vi "press and sound.vi"(9 "stop":bool) -> (10 "frequency":dbl, 11 "data":dbl)   [LabVIEW 2019]
uses:
  <vilib>/sound2/lvsound2.llb/Sound Data Format.ctl
  <vilib>/sound2/lvsound2.llb/Sampling Mode.ctl
  <vilib>/sound2/lvsound2.llb/Sound Output Set Volume (Single).vi
  <vilib>/sound2/lvsound2.llb/Sound Output Write (DBL Single).vi
panel:
  out "0, 1":i16
  out "Array":bool[][](array[boolean])=[[FALSE, FALSE, TRUE, FALSE, FALSE, FALSE, TRUE, FALSE, FALSE, FALSE], [TRUE, TRUE, FALSE, TRUE, FALSE, TRUE, TRUE, FALSE, FALSE, FALSE], [FALSE, TRUE, TRUE, TRUE, FALSE, TRUE, TRUE, FALSE, FALSE, FALSE], [FALSE, FALSE, TRUE, TRUE, TRUE, FALSE, TRUE, FALSE, FALSE, FALSE], [FALSE, TRUE, TRUE, TRUE, TRUE, TRUE, FALSE, FALSE, FALSE, FALSE], [TRUE, TRUE, TRUE, TRUE, TRUE, TRUE, FALSE, FALSE, FALSE, FALSE], [FALSE, FALSE, TRUE, FALSE, FALSE, TRUE, TRUE, TRUE, TRUE, TRUE], [TRUE, TRUE, TRUE, TRUE, TRUE, TRUE, TRUE, TRUE, TRUE, TRUE], [FALSE, TRUE, TRUE, TRUE, TRUE, TRUE, TRUE, TRUE, TRUE, TRUE]]
  in  "stop 4":bool
  out "Boolean":bool
  out "Boolean 5":bool
  out "Boolean 4":bool
  out "Boolean 7":bool
  out "Boolean 6":bool
  out "Boolean 2":bool
  out "Boolean 3":bool
  out "Boolean 8":bool
  out "Boolean 9":bool
  out "Boolean 10":bool
  out "Boolean 11":bool
  out "Boolean 12":bool
  out "Boolean 13":bool
  out "Boolean 14":bool
  out "output array":bool[](array[boolean])
  out "data 8":bool[](array[boolean]) caption="data"
  in  "stop 3":bool
  out "score":dbl
  out "press7":dbl
  out "press6":dbl
  out "press5":dbl
  out "press4":dbl
  out "press3":dbl
  out "press2":dbl
  out "press":dbl
  out "ARDUINO7":dbl
  out "ARDUINO6":dbl
  out "ARDUINO5":dbl
  out "ARDUINO4":dbl
  out "ARDUINO3":dbl
  out "ARDUINO2":dbl
  out "ARDUINO":dbl
  in  "stop (T)":bool=TRUE
  out "data 7":dbl
  out "data 6":dbl
  out "data 5":dbl
  out "data 4":dbl
  out "data 3":dbl
  in  "stop (F) 2":bool caption="stop (F)"
  out "data 2":dbl
  in  "stop 2":bool
  out "Waveform Chart":waveform(dbl)(graph)
  in  "volume":dbl(slide) scale=0.0..100.0
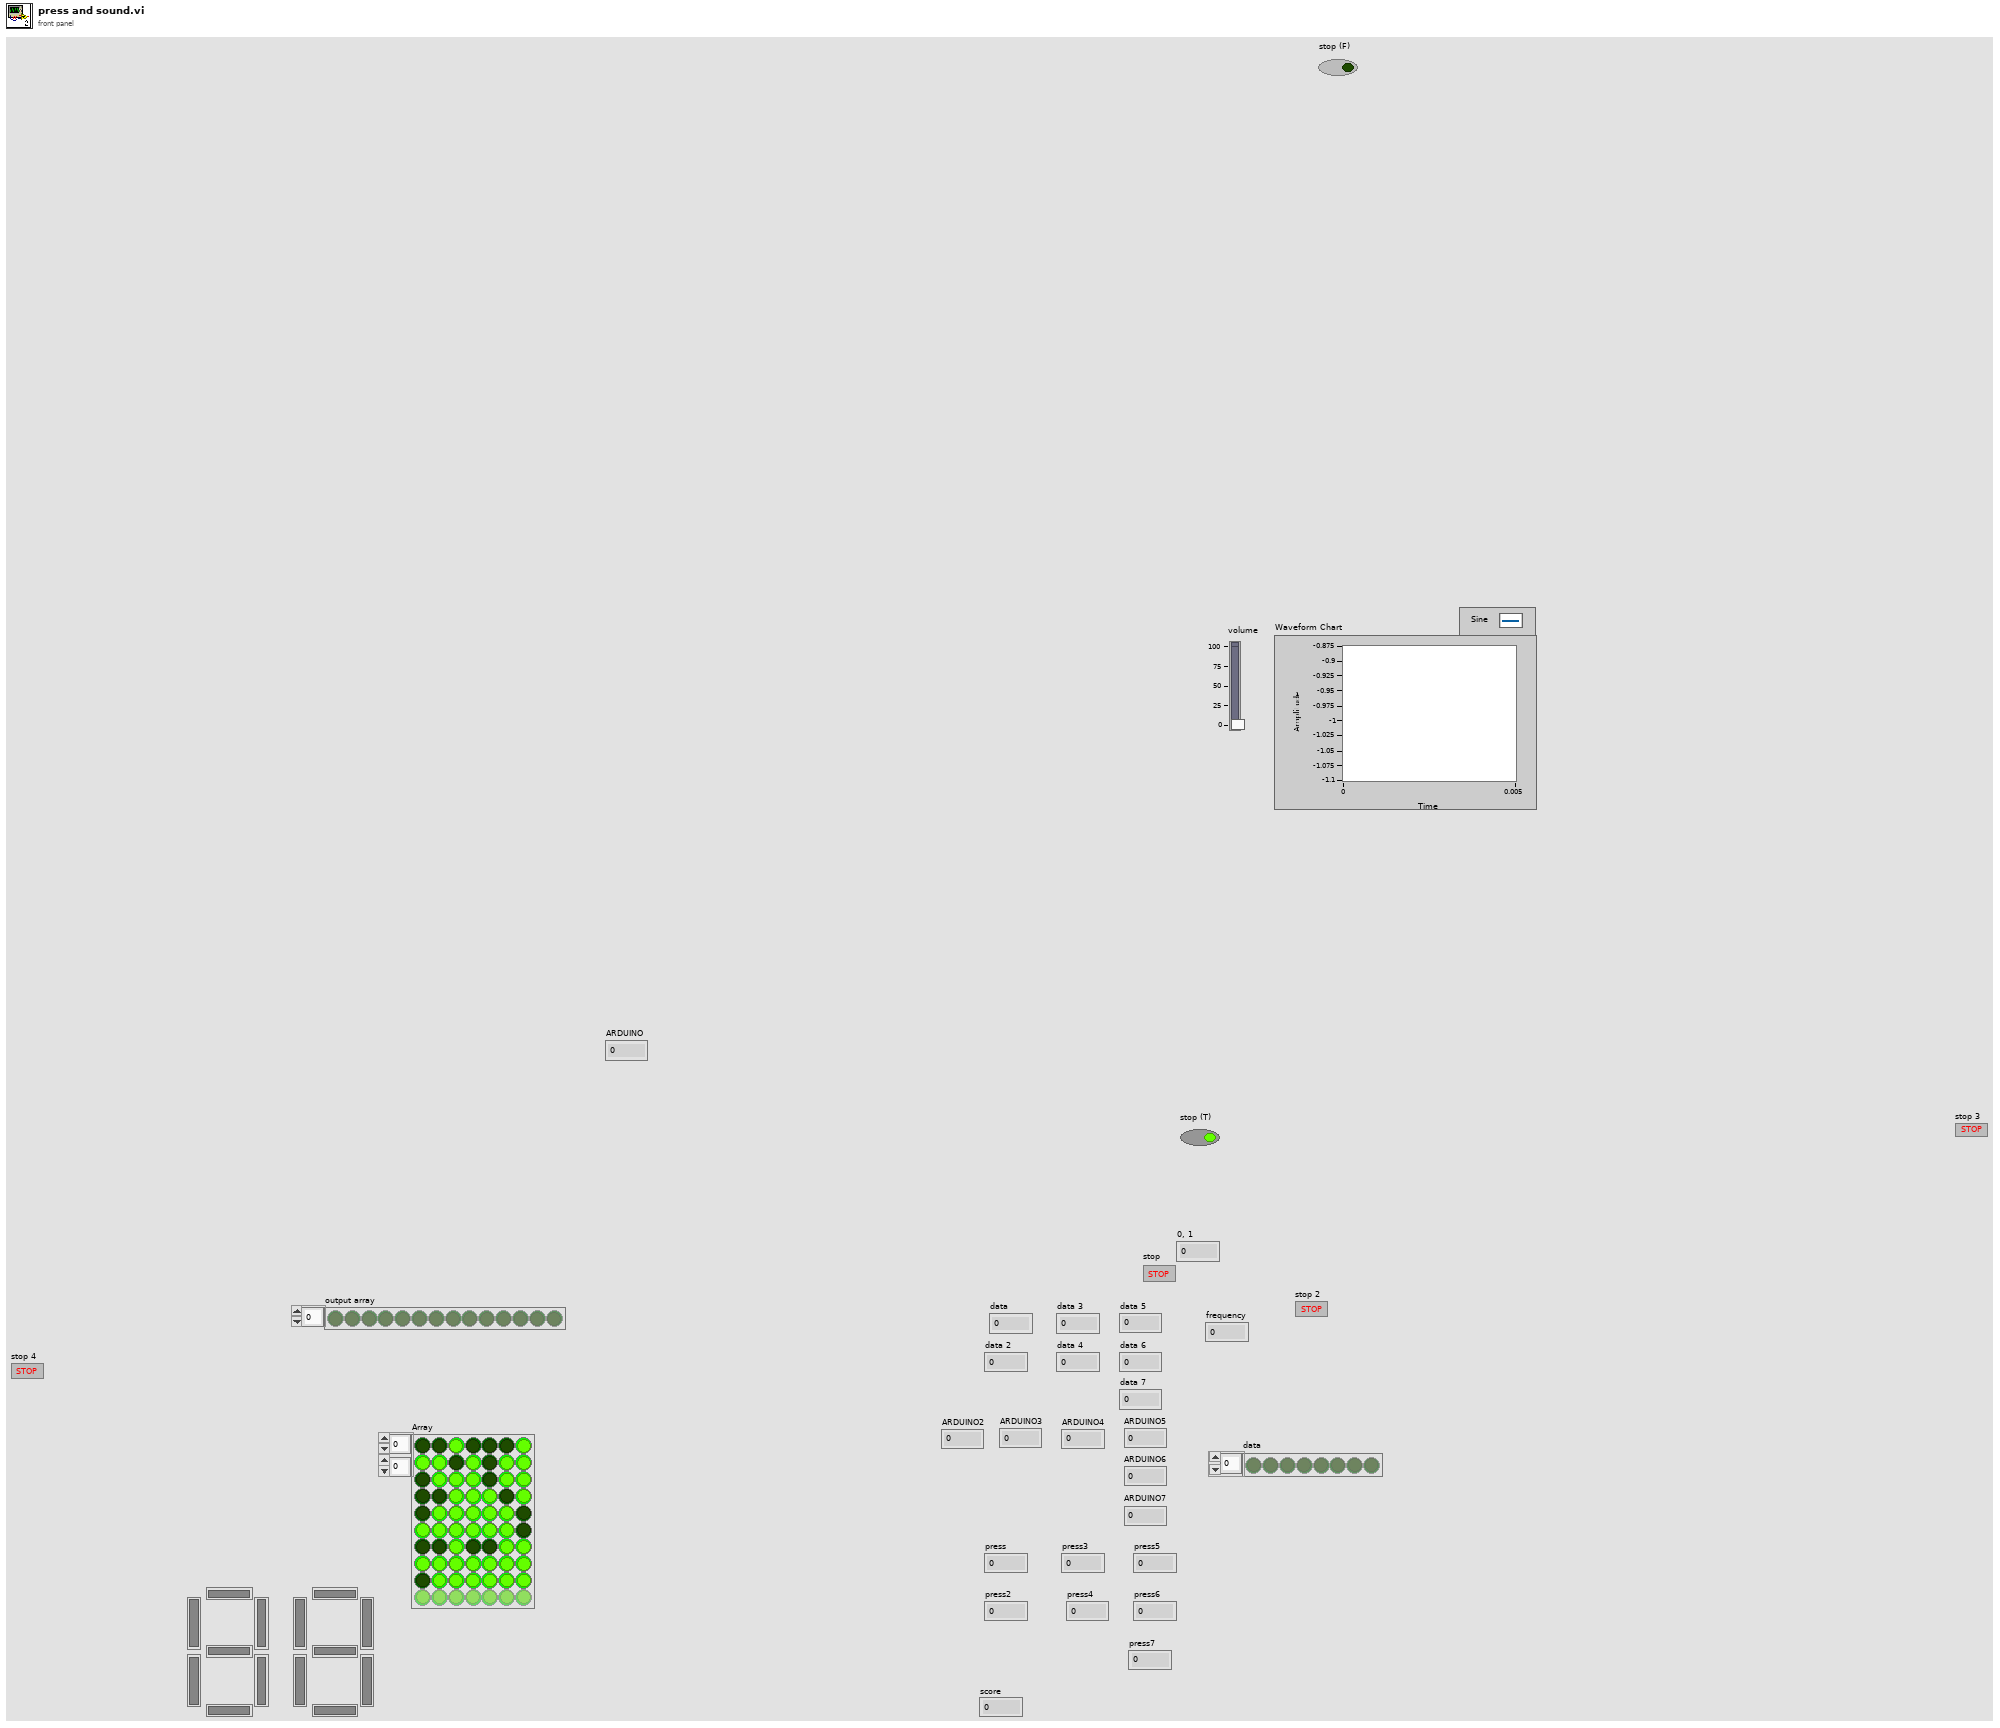
[diagram p1: front panel]
types:
  T1 = typedef "Sampling Mode.ctl" = i32
  T2 = typedef "Sound Data Format.ctl" = cluster{"sample rate (S/s)":dbl, "number of channels":i32, "bits per sample":i32}
  T3 = typedef "Sound Output Task ID.ctl" = u32
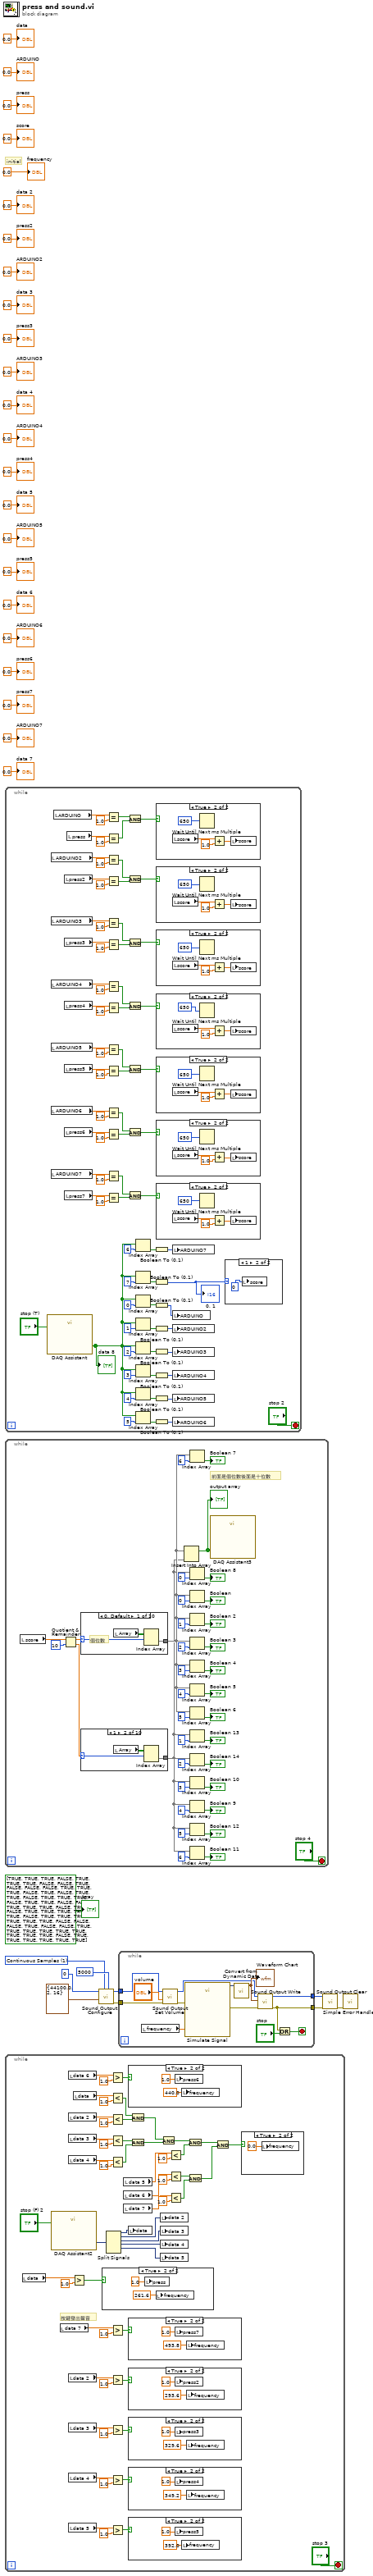
[diagram p0: block diagram]
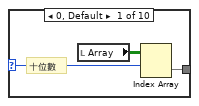
[diagram p2: hidden frame]
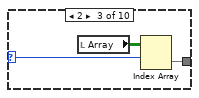
[diagram p3: hidden frame]
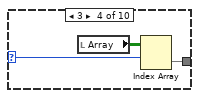
[diagram p4: hidden frame]
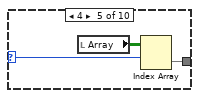
[diagram p5: hidden frame]
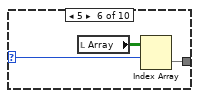
[diagram p6: hidden frame]
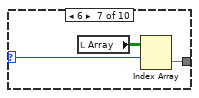
[diagram p7: hidden frame]
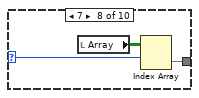
[diagram p8: hidden frame]
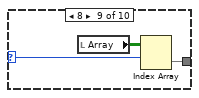
[diagram p9: hidden frame]
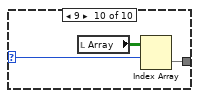
[diagram p10: hidden frame]
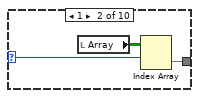
[diagram p11: hidden frame]
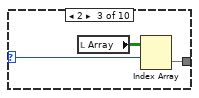
[diagram p12: hidden frame]
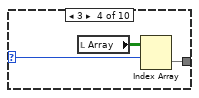
[diagram p13: hidden frame]
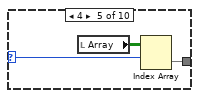
[diagram p14: hidden frame]
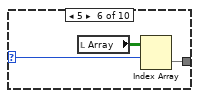
[diagram p15: hidden frame]
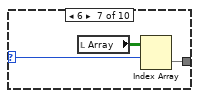
[diagram p16: hidden frame]
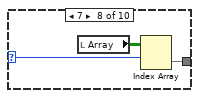
[diagram p17: hidden frame]
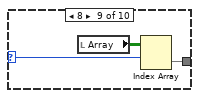
[diagram p18: hidden frame]
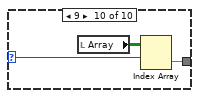
[diagram p19: hidden frame]
diagram:
  w25 = T1 1 items=["Finite Samples", "Continuous Samples"] ("sample mode")
  # "initial"
  n1 = while {
    stop <- "stop 2" stop-if-true
    n2 = call "DAQ Assistant"("stop (T)"="stop (T)") -> ("data"=w36:bool[])  [unwired: 16 in, 2 out]
    "data 8" <- w36
    n3 = local read "ARDUINO2"() -> (w105:dbl)
    n4 = local read "ARDUINO3"() -> (w103:dbl)
    n5 = local read "ARDUINO4"() -> (w101:dbl)
    n6 = local read "ARDUINO5"() -> (w99:dbl)
    n7 = local read "ARDUINO6"() -> (w97:dbl)
    n8 = local read "ARDUINO7"() -> (w95:dbl)
    n9 = local read "ARDUINO"() -> (w107:dbl)
    n10 = local read "press2"() -> (w89:dbl)
    n11 = local read "press3"() -> (w87:dbl)
    n12 = local read "press4"() -> (w85:dbl)
    n13 = local read "press5"() -> (w83:dbl)
    n14 = local read "press6"() -> (w81:dbl)
    n15 = local read "press7"() -> (w79:dbl)
    n16 = local read "press"() -> (w92:dbl)
    n17 = Equal?(x=w107, y=1.0) -> (x = y?=w93:bool)
    n18 = Equal?(x=w92, y=1.0) -> (x = y?=w90:bool)
    n19 = Equal?(x=w105, y=1.0) -> (x = y?=w77:bool)
    n20 = Equal?(x=w89, y=1.0) -> (x = y?=w76:bool)
    n21 = Equal?(x=w103, y=1.0) -> (x = y?=w75:bool)
    n22 = Equal?(x=w87, y=1.0) -> (x = y?=w74:bool)
    n23 = Equal?(x=w101, y=1.0) -> (x = y?=w73:bool)
    n24 = Equal?(x=w85, y=1.0) -> (x = y?=w72:bool)
    n25 = Equal?(x=w99, y=1.0) -> (x = y?=w71:bool)
    n26 = Equal?(x=w83, y=1.0) -> (x = y?=w70:bool)
    n27 = Equal?(x=w97, y=1.0) -> (x = y?=w69:bool)
    n28 = Equal?(x=w81, y=1.0) -> (x = y?=w68:bool)
    n29 = Equal?(x=w95, y=1.0) -> (x = y?=w67:bool)
    n30 = Equal?(x=w79, y=1.0) -> (x = y?=w66:bool)
    n31 = And(x=w93, y=w90) -> (x .and. y?=w65:bool)
    n32 = And(x=w77, y=w76) -> (x .and. y?=w64:bool)
    n33 = And(x=w75, y=w74) -> (x .and. y?=w63:bool)
    n34 = And(x=w73, y=w72) -> (x .and. y?=w62:bool)
    n35 = And(x=w71, y=w70) -> (x .and. y?=w61:bool)
    n36 = And(x=w69, y=w68) -> (x .and. y?=w60:bool)
    n37 = And(x=w67, y=w66) -> (x .and. y?=w59:bool)
    n38 = Index Array(array=w36, index=6) -> (element=w44:bool)
    n39 = Index Array(array=w36, index=7) -> (element=w35:bool)
    n40 = Index Array(array=w36, index=0) -> (element=w50:bool)
    n41 = Index Array(array=w36, index=1) -> (element=w49:bool)
    n42 = Index Array(array=w36, index=2) -> (element=w48:bool)
    n43 = Index Array(array=w36, index=3) -> (element=w47:bool)
    n44 = Index Array(array=w36, index=4) -> (element=w46:bool)
    n45 = Index Array(array=w36, index=5) -> (element=w45:bool)
    n46 = Boolean To (0,1)(Boolean=w44) -> (0, 1=w38:i16)
    n47 = Boolean To (0,1)(Boolean=w35) -> (0, 1=w34:i16)
    "0, 1" <- w34
    n48 = Boolean To (0,1)(Boolean=w50) -> (0, 1=w51:i16)
    n49 = Boolean To (0,1)(Boolean=w49) -> (0, 1=w43:i16)
    n50 = Boolean To (0,1)(Boolean=w48) -> (0, 1=w42:i16)
    n51 = Boolean To (0,1)(Boolean=w47) -> (0, 1=w41:i16)
    n52 = Boolean To (0,1)(Boolean=w46) -> (0, 1=w40:i16)
    n53 = Boolean To (0,1)(Boolean=w45) -> (0, 1=w39:i16)
    n54 = case shown="True" w65 {
      frame False {
      }
      frame True {
        n55 = local read "score"() -> (w138:dbl)
        n56 = Wait Until Next ms Multiple(millisecond multiple=650) -> ()  [unwired: 1 out]
        n57 = Add(x=w138, y=1.0) -> (x+y=w136:dbl)
        n58 = local write "score"(w136) -> ()
      }
    }
    n59 = case shown="True" w64 {
      frame False {
      }
      frame True {
        n60 = local read "score"() -> (w134:dbl)
        n61 = Wait Until Next ms Multiple(millisecond multiple=650) -> ()  [unwired: 1 out]
        n62 = Add(x=w134, y=1.0) -> (x+y=w132:dbl)
        n63 = local write "score"(w132) -> ()
      }
    }
    n64 = case shown="True" w63 {
      frame False {
      }
      frame True {
        n65 = local read "score"() -> (w130:dbl)
        n66 = Wait Until Next ms Multiple(millisecond multiple=650) -> ()  [unwired: 1 out]
        n67 = Add(x=w130, y=1.0) -> (x+y=w128:dbl)
        n68 = local write "score"(w128) -> ()
      }
    }
    n69 = case shown="True" w62 {
      frame False {
      }
      frame True {
        n70 = local read "score"() -> (w126:dbl)
        n71 = Wait Until Next ms Multiple(millisecond multiple=650) -> ()  [unwired: 1 out]
        n72 = Add(x=w126, y=1.0) -> (x+y=w124:dbl)
        n73 = local write "score"(w124) -> ()
      }
    }
    n74 = case shown="True" w61 {
      frame False {
      }
      frame True {
        n75 = local read "score"() -> (w122:dbl)
        n76 = Wait Until Next ms Multiple(millisecond multiple=650) -> ()  [unwired: 1 out]
        n77 = Add(x=w122, y=1.0) -> (x+y=w120:dbl)
        n78 = local write "score"(w120) -> ()
      }
    }
    n79 = case shown="True" w60 {
      frame False {
      }
      frame True {
        n80 = local read "score"() -> (w118:dbl)
        n81 = Wait Until Next ms Multiple(millisecond multiple=650) -> ()  [unwired: 1 out]
        n82 = Add(x=w118, y=1.0) -> (x+y=w116:dbl)
        n83 = local write "score"(w116) -> ()
      }
    }
    n84 = case shown="True" w59 {
      frame False {
      }
      frame True {
        n85 = local read "score"() -> (w114:dbl)
        n86 = Wait Until Next ms Multiple(millisecond multiple=650) -> ()  [unwired: 1 out]
        n87 = Add(x=w114, y=1.0) -> (x+y=w112:dbl)
        n88 = local write "score"(w112) -> ()
      }
    }
    n89 = local write "ARDUINO7"(w38) -> ()
    n90 = local write "ARDUINO"(w51) -> ()
    n91 = local write "ARDUINO2"(w43) -> ()
    n92 = local write "ARDUINO3"(w42) -> ()
    n93 = local write "ARDUINO4"(w41) -> ()
    n94 = local write "ARDUINO5"(w40) -> ()
    n95 = local write "ARDUINO6"(w39) -> ()
    n96 = case shown="1" w34 {
      frame 0, Default {
      }
      frame 1 {
        n97 = local write "score"(0) -> ()
      }
    }
  }
  n98 = while {
    stop <- "stop 4" stop-if-true
    # "前面是個位數後面是十位數"
    n99 = local read "score"() -> (w139:dbl)
    n100 = Quotient & Remainder(x=w139, y=10) -> (x-y*floor(x/y)=w142:dbl, floor(x/y)=w141:dbl)
    n101 = case shown="0, Default" w142 {
      selector: w142 -> [w205 w209 w212 w215 w218 w221 w224 w227 w230 w233]
      tunnel: [w206 w208 w211 w214 w217 w220 w223 w226 w229 w232] -> w144
      frame 0, Default {
        # "個位數"
        n102 = local read "Array"() -> (w207:bool[][])
        n103 = Index Array(array=w207, index (row)=w205) -> (element=w206:bool[])  [unwired: 1 in]
      }
      frame 1 {
        n104 = local read "Array"() -> (w210:bool[][])
        n105 = Index Array(array=w210, index (row)=w209) -> (element=w208:bool[])  [unwired: 1 in]
      }
      frame 2 {
        n106 = local read "Array"() -> (w213:bool[][])
        n107 = Index Array(array=w213, index (row)=w212) -> (element=w211:bool[])  [unwired: 1 in]
      }
      frame 3 {
        n108 = local read "Array"() -> (w216:bool[][])
        n109 = Index Array(array=w216, index (row)=w215) -> (element=w214:bool[])  [unwired: 1 in]
      }
      frame 4 {
        n110 = local read "Array"() -> (w219:bool[][])
        n111 = Index Array(array=w219, index (row)=w218) -> (element=w217:bool[])  [unwired: 1 in]
      }
      frame 5 {
        n112 = local read "Array"() -> (w222:bool[][])
        n113 = Index Array(array=w222, index (row)=w221) -> (element=w220:bool[])  [unwired: 1 in]
      }
      frame 6 {
        n114 = local read "Array"() -> (w225:bool[][])
        n115 = Index Array(array=w225, index (row)=w224) -> (element=w223:bool[])  [unwired: 1 in]
      }
      frame 7 {
        n116 = local read "Array"() -> (w228:bool[][])
        n117 = Index Array(array=w228, index (row)=w227) -> (element=w226:bool[])  [unwired: 1 in]
      }
      frame 8 {
        n118 = local read "Array"() -> (w231:bool[][])
        n119 = Index Array(array=w231, index (row)=w230) -> (element=w229:bool[])  [unwired: 1 in]
      }
      frame 9 {
        n120 = local read "Array"() -> (w234:bool[][])
        n121 = Index Array(array=w234, index (row)=w233) -> (element=w232:bool[])  [unwired: 1 in]
      }
    }
    n122 = case shown="1" w141 {
      selector: w141 -> [w175 w179 w183 w186 w189 w192 w195 w198 w201 w204]
      tunnel: [w176 w178 w181 w184 w187 w190 w193 w196 w199 w202] -> w143
      frame 0, Default {
        # "十位數"
        n123 = local read "Array"() -> (w177:bool[][])
        n124 = Index Array(array=w177, index (row)=w175) -> (element=w176:bool[])  [unwired: 1 in]
      }
      frame 1 {
        n125 = local read "Array"() -> (w180:bool[][])
        n126 = Index Array(array=w180, index (row)=w179) -> (element=w178:bool[])  [unwired: 1 in]
      }
      frame 2 {
        n127 = local read "Array"() -> (w182:bool[][])
        n128 = Index Array(array=w182, index (row)=w183) -> (element=w181:bool[])  [unwired: 1 in]
      }
      frame 3 {
        n129 = local read "Array"() -> (w185:bool[][])
        n130 = Index Array(array=w185, index (row)=w186) -> (element=w184:bool[])  [unwired: 1 in]
      }
      frame 4 {
        n131 = local read "Array"() -> (w188:bool[][])
        n132 = Index Array(array=w188, index (row)=w189) -> (element=w187:bool[])  [unwired: 1 in]
      }
      frame 5 {
        n133 = local read "Array"() -> (w191:bool[][])
        n134 = Index Array(array=w191, index (row)=w192) -> (element=w190:bool[])  [unwired: 1 in]
      }
      frame 6 {
        n135 = local read "Array"() -> (w194:bool[][])
        n136 = Index Array(array=w194, index (row)=w195) -> (element=w193:bool[])  [unwired: 1 in]
      }
      frame 7 {
        n137 = local read "Array"() -> (w197:bool[][])
        n138 = Index Array(array=w197, index (row)=w198) -> (element=w196:bool[])  [unwired: 1 in]
      }
      frame 8 {
        n139 = local read "Array"() -> (w200:bool[][])
        n140 = Index Array(array=w200, index (row)=w201) -> (element=w199:bool[])  [unwired: 1 in]
      }
      frame 9 {
        n141 = local read "Array"() -> (w203:bool[][])
        n142 = Index Array(array=w203, index (row)=w204) -> (element=w202:bool[])  [unwired: 1 in]
      }
    }
    n143 = Insert Into Array(array=w144, new element=w143) -> (w140:bool[])  [unwired: 1 in]
    "output array" <- w140
    n144 = Index Array(array=w144, index=6) -> (element=→"Boolean 7":bool)
    n145 = Index Array(array=w143, index=0) -> (element=→"Boolean 8":bool)
    n146 = Index Array(array=w144, index=0) -> (element=→"Boolean":bool)
    n147 = Index Array(array=w144, index=1) -> (element=→"Boolean 2":bool)
    n148 = Index Array(array=w144, index=2) -> (element=→"Boolean 3":bool)
    n149 = Index Array(array=w144, index=3) -> (element=→"Boolean 4":bool)
    n150 = Index Array(array=w144, index=4) -> (element=→"Boolean 5":bool)
    n151 = Index Array(array=w144, index=5) -> (element=→"Boolean 6":bool)
    n152 = Index Array(array=w143, index=1) -> (element=→"Boolean 13":bool)
    n153 = Index Array(array=w143, index=2) -> (element=→"Boolean 14":bool)
    n154 = Index Array(array=w143, index=3) -> (element=→"Boolean 10":bool)
    n155 = Index Array(array=w143, index=4) -> (element=→"Boolean 9":bool)
    n156 = Index Array(array=w143, index=5) -> (element=→"Boolean 12":bool)
    n157 = Index Array(array=w143, index=6) -> (element=→"Boolean 11":bool)
    n158 = call "DAQ Assistant3"("data"=w140) -> ()  [unwired: 17 in, 2 out]
  }
  n159 = while {
    stop <- "stop 3" stop-if-true
    # "按鍵發出聲音"
    n160 = local read "data"() -> (w288:dbl)
    n161 = call "DAQ Assistant2"("stop (T)"="stop (F) 2") -> ("data"=w267:dynamicdata)  [unwired: 16 in, 2 out]
    n162 = local read "data 7"() -> (w274:dbl)
    n163 = local read "data 6"() -> (w275:dbl)
    n164 = local read "data 2"() -> (w249:dbl)
    n165 = local read "data 3"() -> (w247:dbl)
    n166 = local read "data 4"() -> (w245:dbl)
    n167 = local read "data 2"() -> (w287:dbl)
    n168 = local read "data 3"() -> (w283:dbl)
    n169 = local read "data 4"() -> (w282:dbl)
    n170 = local read "data 5"() -> (w277:dbl)
    n171 = Greater?(x=w288, y=1.0) -> (0:w289:bool)
    n172 = local read "data"() -> (w251:dbl)
    n173 = case shown="True" w289 {
      frame False {
        n174 = local write "press"(0.0 ("ARDUINO")) -> ()
      }
      frame True {
        n175 = local write "press"(1.0 ("ARDUINO")) -> ()
        n176 = local write "frequency"(261.6 ("frequency")) -> ()
      }
    }
    n177 = Split Signals(w267) -> (w266:dynamicdata, w265:dynamicdata, w264:dynamicdata, w263:dynamicdata, w262:dynamicdata)  [unwired: 6 in, 1 out]
    n178 = Greater?(x=w275, y=1.0) -> (0:w271:bool)
    n179 = Less?(x=w251, y=1.0) -> (x < y?=w250:bool)
    n180 = Less?(x=w249, y=1.0) -> (x < y?=w248:bool)
    n181 = Less?(x=w247, y=1.0) -> (x < y?=w246:bool)
    n182 = Less?(x=w245, y=1.0) -> (x < y?=w244:bool)
    n183 = Greater?(x=w274, y=1.0) -> (0:w270:bool)
    n184 = Greater?(x=w287, y=1.0) -> (0:w286:bool)
    n185 = Greater?(x=w283, y=1.0) -> (0:w284:bool)
    n186 = Greater?(x=w282, y=1.0) -> (0:w280:bool)
    n187 = Greater?(x=w277, y=1.0) -> (0:w278:bool)
    n188 = local read "data 5"() -> (w243:dbl)
    n189 = local read "data 6"() -> (w241:dbl)
    n190 = local read "data 7"() -> (w240:dbl)
    n191 = case shown="True" w271 {
      frame False {
        n192 = local write "press6"(0.0 ("ARDUINO6")) -> ()
      }
      frame True {
        n193 = local write "press6"(1.0 ("ARDUINO6")) -> ()
        n194 = local write "frequency"(440.0 ("frequency")) -> ()
      }
    }
    n195 = local write "data"(w266) -> ()
    n196 = case shown="True" w270 {
      frame False {
        n197 = local write "press7"(0.0 ("ARDUINO7")) -> ()
      }
      frame True {
        n198 = local write "press7"(1.0 ("ARDUINO7")) -> ()
        n199 = local write "frequency"(493.8 ("frequency")) -> ()
      }
    }
    n200 = case shown="True" w286 {
      frame False {
        n201 = local write "press2"(0.0 ("ARDUINO2")) -> ()
      }
      frame True {
        n202 = local write "press2"(1.0 ("ARDUINO2")) -> ()
        n203 = local write "frequency"(293.6 ("frequency")) -> ()
      }
    }
    n204 = case shown="True" w284 {
      frame False {
        n205 = local write "press3"(0.0 ("ARDUINO3")) -> ()
      }
      frame True {
        n206 = local write "press3"(1.0 ("ARDUINO3")) -> ()
        n207 = local write "frequency"(329.6 ("frequency")) -> ()
      }
    }
    n208 = case shown="True" w280 {
      frame False {
        n209 = local write "press4"(0.0 ("ARDUINO4")) -> ()
      }
      frame True {
        n210 = local write "press4"(1.0 ("ARDUINO4")) -> ()
        n211 = local write "frequency"(349.2 ("frequency")) -> ()
      }
    }
    n212 = case shown="True" w278 {
      frame False {
        n213 = local write "press5"(0.0 ("ARDUINO5")) -> ()
      }
      frame True {
        n214 = local write "press5"(1.0 ("ARDUINO5")) -> ()
        n215 = local write "frequency"(392.0 ("frequency")) -> ()
      }
    }
    n216 = And(x=w250, y=w248) -> (x .and. y?=w254:bool)
    n217 = And(x=w246, y=w244) -> (x .and. y?=w253:bool)
    n218 = local write "data 2"(w265) -> ()
    n219 = local write "data 3"(w264) -> ()
    n220 = local write "data 4"(w263) -> ()
    n221 = local write "data 5"(w262) -> ()
    n222 = And(x=w254, y=w253) -> (x .and. y?=w252:bool)
    n223 = Less?(x=w243, y=1.0) -> (x < y?=w242:bool)
    n224 = Less?(x=w241, y=1.0) -> (x < y?=w239:bool)
    n225 = Less?(x=w240, y=1.0) -> (x < y?=w238:bool)
    n226 = And(x=w252, y=w242) -> (x .and. y?=w236:bool)
    n227 = And(x=w239, y=w238) -> (x .and. y?=w237:bool)
    n228 = And(x=w236, y=w237) -> (x .and. y?=w235:bool)
    n229 = case shown="True" w235 {
      frame False {
      }
      frame True {
        n230 = local write "frequency"(0.0 ("frequency")) -> ()
      }
    }
  }
  n231 = call <vilib>:"Sound Output Configure.vi"("number of samples/ch"=5000, "sample mode"=w25, "sound format"=T2 {"sample rate (S/s)"=44100.0, "number of channels"=2, "bits per sample"=16}, "device ID"=u32 0) -> ("error out"=w31:errorcluster, "task ID"=w30:T3)  [unwired: 6 in]
  n232 = while {
    tunnel: w31 -> [w323]
    tunnel: w30 -> [w321]
    tunnel: [w315] -> w28
    tunnel: [w314] -> w29
    stop <- w324 stop-if-true
    n233 = local read "frequency"() -> (w313:dbl)
    n234 = call-poly <vilib>:"Sound Output Set Volume.vi"("error in (no error)"=w323, "volume"="volume", "task ID"=w321) -> ("error out"=w320:errorcluster, "task ID out"=w316:T3)  [unwired: 7 in]
    n235 = call "Simulate Signal"("Frequency"=w313, "error in (no error)"=w320) -> ("Sine"=w319:dynamicdata, "error out"=w318:errorcluster)  [unwired: 12 in]
    n236 = call "Convert from Dynamic Data"("Dynamic Data Type"=w319) -> ("Waveform"=w317:waveform(dbl))  [unwired: 3 in]
    "Waveform Chart" <- w317
    n237 = call-poly <vilib>:"Sound Output Write.vi"("error in (no error)"=w318, "data"=w317, "task ID"=w316) -> ("error out"=w315:errorcluster, "task ID out"=w314:T3)  [unwired: 7 in]
    n238 = Or(x=w315, y="stop") -> (x .or. y?=w324:bool)
  }
  n239 = call <vilib>:"Sound Output Clear.vi"("error in (no error)"=w28, "task ID"=w29) -> ("error out"=w27:errorcluster)  [unwired: 9 in]
  n240 = call <vilib>:"Simple Error Handler.vi"("error in (no error)"=w27) -> ()  [unwired: 4 in, 5 out]
  "frequency" <- 0.0 ("frequency")
  "data" <- 0.0 ("data")
  "data 2" <- 0.0 ("data")
  "data 3" <- 0.0 ("data")
  "data 4" <- 0.0 ("data")
  "data 5" <- 0.0 ("data")
  "data 6" <- 0.0 ("data")
  "data 7" <- 0.0 ("data")
  "ARDUINO5" <- 0.0 ("ARDUINO5")
  "ARDUINO6" <- 0.0 ("ARDUINO6")
  "ARDUINO3" <- 0.0 ("ARDUINO3")
  "ARDUINO2" <- 0.0 ("ARDUINO2")
  "ARDUINO4" <- 0.0 ("ARDUINO4")
  "ARDUINO7" <- 0.0 ("ARDUINO7")
  "ARDUINO" <- 0.0 ("ARDUINO")
  "press" <- 0.0 ("press")
  "press3" <- 0.0 ("press3")
  "press5" <- 0.0 ("press5")
  "press2" <- 0.0 ("press2")
  "press4" <- 0.0 ("press4")
  "press6" <- 0.0 ("press6")
  "press7" <- 0.0 ("press7")
  "score" <- 0.0 ("score")
  "Array" <- bool[][] [[TRUE, TRUE, TRUE, FALSE, TRUE, TRUE, TRUE], [FALSE, FALSE, TRUE, FALSE, FALSE, FALSE, TRUE], [TRUE, TRUE, FALSE, TRUE, FALSE, TRUE, TRUE], [FALSE, TRUE, TRUE, TRUE, FALSE, TRUE, TRUE], [FALSE, FALSE, TRUE, TRUE, TRUE, FALSE, TRUE], [FALSE, TRUE, TRUE, TRUE, TRUE, TRUE, FALSE], [TRUE, TRUE, TRUE, TRUE, TRUE, TRUE, FALSE], [FALSE, FALSE, TRUE, FALSE, FALSE, TRUE, TRUE], [TRUE, TRUE, TRUE, TRUE, TRUE, TRUE, TRUE], [FALSE, TRUE, TRUE, TRUE, TRUE, TRUE, TRUE]]
